vi "Exchange Main Camera.vi"(8 "error in (no error)":errorcluster, 10 "New Main Cam":string, 11 "HIJ 4 Alignment Cams App in":refnum<class "HIJ 3 Alignment Cams App.lvclass">) -> (0 "error out":errorcluster, 3 "HIJ 4 Alignment Cams App out":refnum<class "HIJ 3 Alignment Cams App.lvclass">)   [LabVIEW 2014, in "HIJ 3 Alignment Cams App.lvlib" / "HIJ 3 Alignment Cams App.lvclass"]
uses:
  HIJ 3 Alignment Cams App.lvclass
  HIJ 3 Alignment Cams App.lvclass/HIJ 3 Alignment Cams App.ctl
  <vilib>/ActorFramework/Message Enqueuer/Message Priority.ctl
  <vilib>/ActorFramework/Message Enqueuer/Message Enqueuer.lvclass/Message Enqueuer.ctl
  Viewable Actor/ViewableActor Messages/Insert Into SubPanel Msg/Insert Into SubPanel Msg.lvclass/Insert Into SubPanel Msg.ctl
  <vilib>/ActorFramework/Message Enqueuer/Enqueue.vi
  <vilib>/ActorFramework/Message Priority Queue/Priority Enqueue.vi
  Viewable Actor/ViewableActor Messages/Remove From SubPanel Msg/Remove From SubPanel Msg.lvclass
  Viewable Actor/ViewableActor Messages/Insert Into SubPanel Msg/Insert Into SubPanel Msg.lvclass
  <vilib>/ActorFramework/Message Enqueuer/Message Enqueuer.lvclass
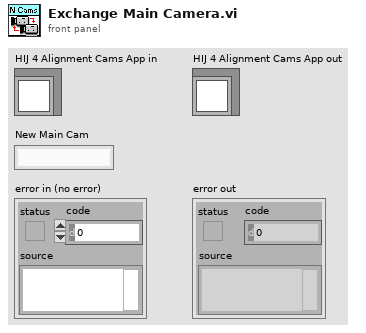
[diagram p1: front panel]
types:
  T1 = typedef "HIJ 3 Alignment Cams App.lvlib/HIJ 3 Alignment Cams App.lvclass/CamAppInfo.ctl" = cluster{"Camera":T2, "App enq":refnum<class "Message Enqueuer.lvclass">, "SubPnl Refnum":refnum<vi>}
  T2 = typedef "IMAQdx.ctl" = refnum<k21>
  T3 = typedef "Actor Framework.lvlib/Message Enqueuer.lvclass/Message Priority.ctl" = enum16{"Low", "Normal", "High"}
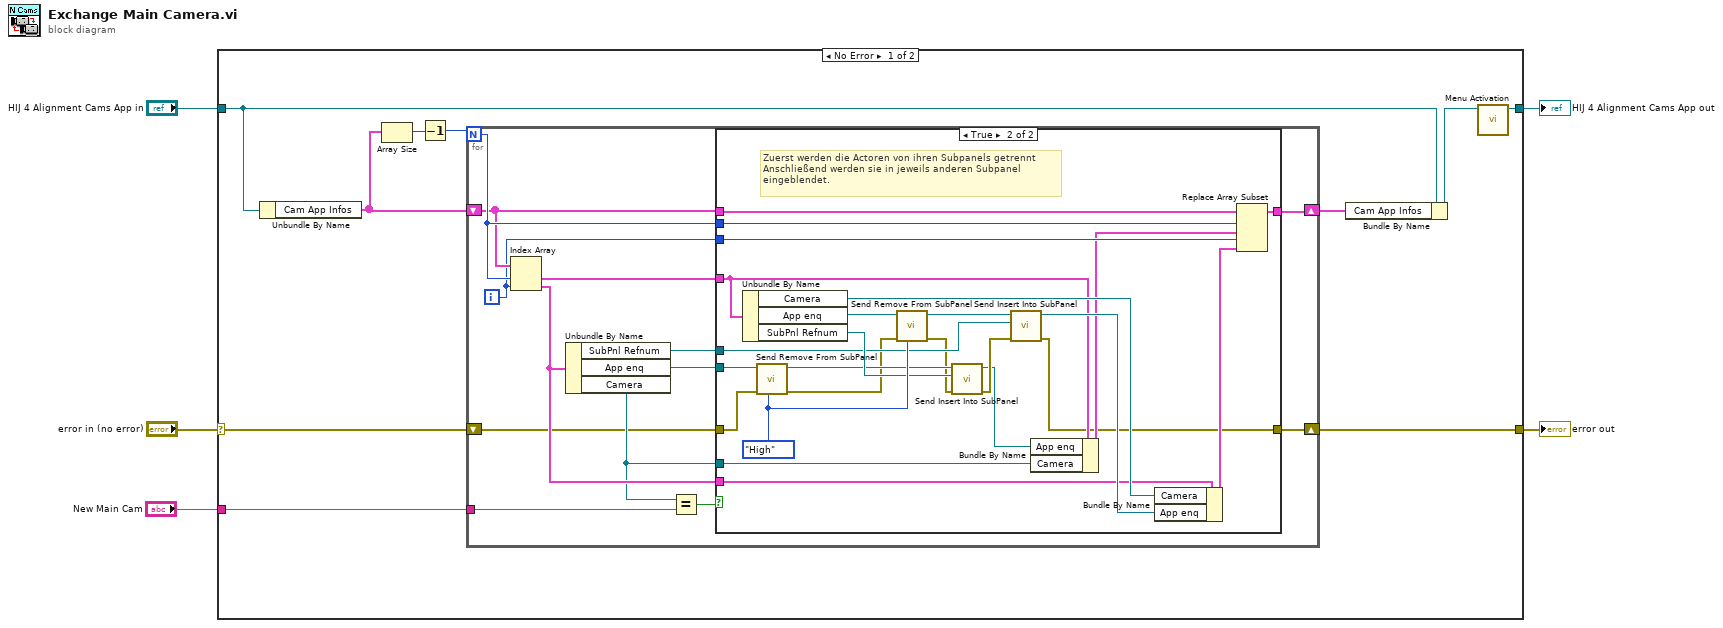
[diagram p0: block diagram]
diagram:
  n1 = case shown="No Error" "error in (no error)" {
    selector: "error in (no error)" -> [w11 w56]
    tunnel: [w10 w56] -> w4
    tunnel: [w7 w55] -> w2
    tunnel: "HIJ 4 Alignment Cams App in" -> [w6 w55]
    tunnel: "New Main Cam" -> [w15 _]
    frame No Error {
      n2 = Unbundle By Name(w6) -> ("Cam App Infos"=w14:T1[])
      n3 = Array Size(array=w14) -> (size(s)=w13:i32)
      n4 = Decrement(x=w13) -> (x-1=w12:i32)
      n5 = for {
        N: w12 -> [w28]
        tunnel: w15 -> [w27]
        shift-right: [w22] -> w9
        shift-left: w14 -> [w25]
        shift-right: [w16] -> w10
        shift-left: w11 -> [w17]
        i -> [w20]
        n6 = Index Array(array=w25, index #1=w28, index #2=w20) -> (element #1=w24:T1, element #2=w19:T1)
        n7 = Unbundle By Name(w19) -> ("SubPnl Refnum"=w21:refnum<vi>, "App enq"=w23:refnum<class "Message Enqueuer.lvclass">, "Camera"=w18:T2)
        n8 = Equal?(x=w18, y=w27) -> (x = y?=w26:bool)
        n9 = case shown="True" w26 {
          tunnel: w25 -> [w30 w49]
          tunnel: w24 -> [_ w42]
          tunnel: w23 -> [_ w48]
          tunnel: [w30 w45] -> w22
          tunnel: w21 -> [_ w44]
          tunnel: w20 -> [_ w53]
          tunnel: w28 -> [_ w37]
          tunnel: w19 -> [_ w35]
          tunnel: w18 -> [_ w36]
          tunnel: w17 -> [w29 w33]
          tunnel: [w29 w32] -> w16
          frame False {
          }
          frame True {
            w51 = Message_Priority."High" ("Message Priority (Normal)")
            # "Zuerst werden die Actoren von ihren Subpanels getrennt\nAnschließend werden sie in jeweils anderen Subpanel\neingeblendet."
            n10 = Unbundle By Name(w42) -> ("Camera"=w52:T2, "App enq"=w47:refnum<class "Message Enqueuer.lvclass">, "SubPnl Refnum"=w50:refnum<vi>)
            n11 = call "Send Remove From SubPanel.vi"("Message Priority (Normal)"=w51, "error in (no error)"=w33, "Message Enqueuer"=w48) -> ("error out"=w40:errorcluster, "Message Enqueuer out"=w46:refnum<class "Message Enqueuer.lvclass">)  [unwired: 7 in]
            n12 = call "Send Remove From SubPanel.vi"("Message Priority (Normal)"=w51, "error in (no error)"=w40, "Message Enqueuer"=w47) -> ("error out"=w39:errorcluster, "Message Enqueuer out"=w43:refnum<class "Message Enqueuer.lvclass">)  [unwired: 7 in]
            n13 = call "Send Insert Into SubPanel.vi"("error in (no error)"=w39, "SubPanel Ref"=w50, "Message Enqueuer"=w46) -> ("error out"=w38:errorcluster, "Message Enqueuer out"=w31:refnum<class "Message Enqueuer.lvclass">)  [unwired: 7 in]
            n14 = call "Send Insert Into SubPanel.vi"("error in (no error)"=w38, "SubPanel Ref"=w44, "Message Enqueuer"=w43) -> ("error out"=w32:errorcluster, "Message Enqueuer out"=w54:refnum<class "Message Enqueuer.lvclass">)  [unwired: 7 in]
            n15 = Bundle By Name(cluster=w42, "App enq"=w31, "Camera"=w36) -> (w41:T1)
            n16 = Bundle By Name(cluster=w35, "Camera"=w52, "App enq"=w54) -> (w34:T1)
            n17 = Replace Array Subset(array=w49, new element #1=w41, index #1=w37, new element #2=w34, index #2=w53) -> (w45:T1[])
          }
        }
      }
      n18 = Bundle By Name(cluster=w6, "Cam App Infos"=w9) -> (w8:refnum<class "HIJ 3 Alignment Cams App.lvclass">)
      n19 = call "Menu Activation.vi"("HIJ 4 Alignment Cams App in"=w8) -> ("HIJ 4 Alignment Cams App out"=w7:refnum<class "HIJ 3 Alignment Cams App.lvclass">)  [unwired: 9 in, 1 out]
    }
    frame Error {
    }
  }
  "error out" <- w4
  "HIJ 4 Alignment Cams App out" <- w2
